vi "ReadExcel.vi"(1 "读出文本":bool, 2 "导出sheet位号":i8=1, 3 "路径":path) -> (0 "EXCEL读取":string[][](array[string]))   [LabVIEW 2011]
panel:
  in  "Excel._Worksheet":refnum<k7>
  in  "Excel._Application":refnum<k7>
  # "将对应路径 Excel 中的表格数据转换为数组数据"
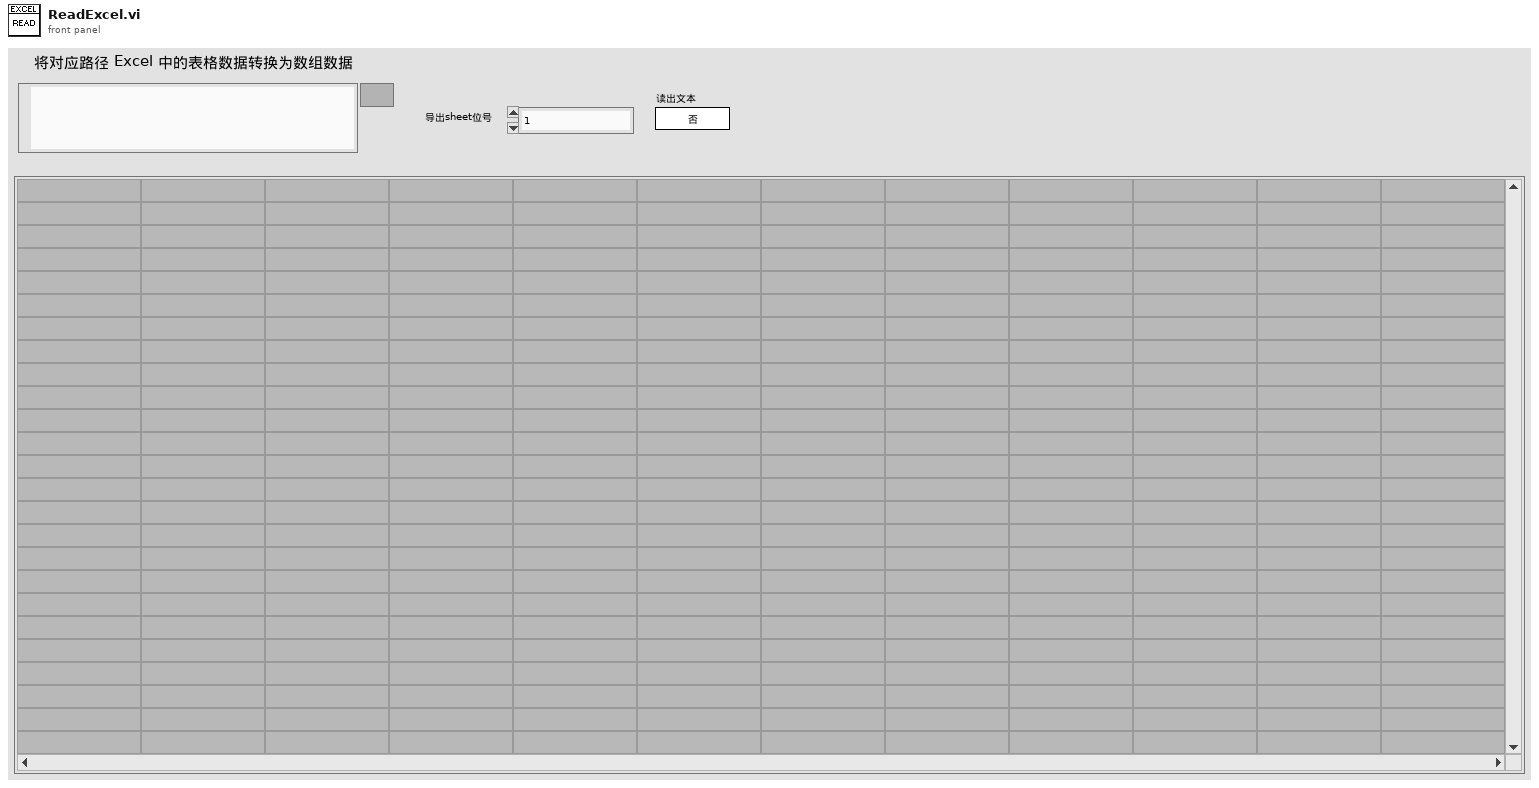
[diagram p1: front panel]
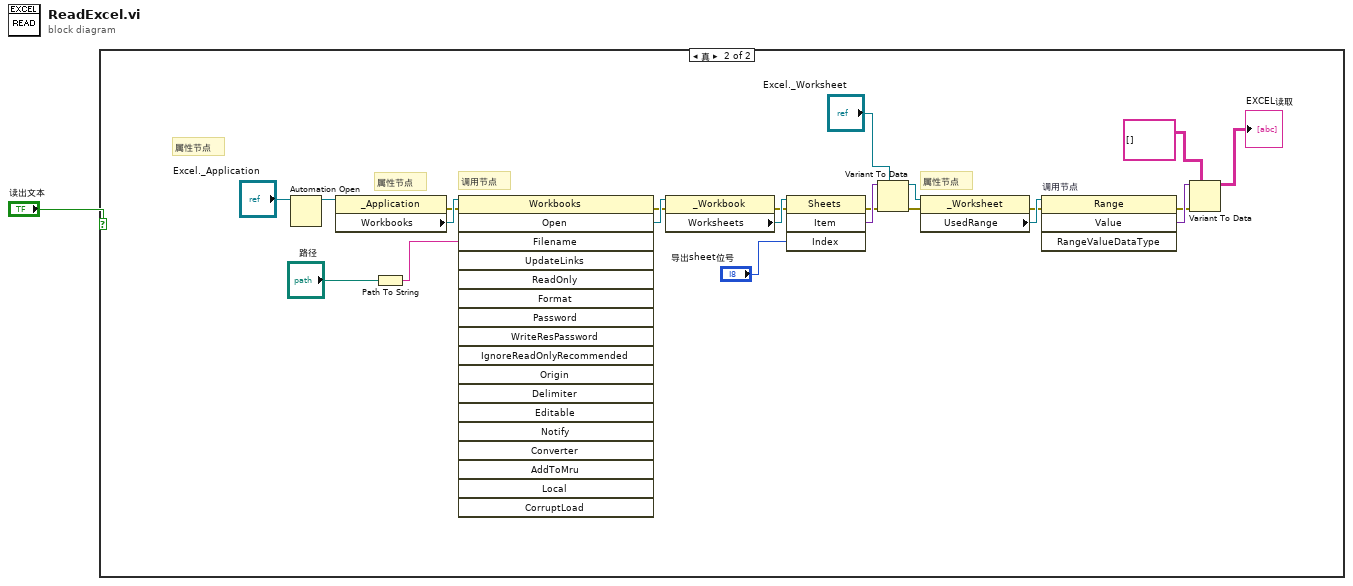
[diagram p0: block diagram]
diagram:
  n1 = case shown="真" "读出文本" {
    frame False {
    }
    frame True {
      # "属性节点"
      # "属性节点"
      # "属性节点"
      # "调用节点"
      n2 = Automation Open(Automation Refnum="Excel._Application") -> (Automation Refnum=w21:refnum<k7>)  [unwired: 3 in, 1 out]
      n3 = property class="_Application"(reference=w21) -> (error out=w19:errorcluster, "Workbooks"=w20:refnum<k7>)  [unwired: 1 in, 1 out]
      n4 = Path To String(path="路径") -> (string=w2:string)
      n5 = invoke class="Workbooks" method="Open"(reference=w20, error in=w19, "Filename"=w2) -> (error out=w17:errorcluster, "Open"=w18:refnum<k7>)  [unwired: 15 in, 16 out]
      n6 = property class="_Workbook"(reference=w18, error in=w17) -> (error out=w14:errorcluster, "Worksheets"=w15:refnum<k7>)  [unwired: 1 out]
      n7 = invoke class="Sheets" method="Item"(reference=w15, error in=w14, "Index"="导出sheet位号") -> (error out=w12:errorcluster, "Item"=w13:variant)  [unwired: 1 in, 2 out]
      n8 = Variant To Data(error in=w12, type="Excel._Worksheet", Variant=w13) -> (data=w10:refnum<k7>, error out=w9:errorcluster)
      n9 = property class="_Worksheet"(reference=w10, error in=w9) -> (error out=w7:errorcluster, "UsedRange"=w8:refnum<k7>)  [unwired: 1 out]
      n10 = invoke on="调用节点" class="Range" method="Value"(reference=w8, error in=w7) -> (error out=w5:errorcluster, "Value"=w6:variant)  [unwired: 2 in, 2 out]
      n11 = Variant To Data(error in=w5, type=string[][] [], Variant=w6) -> (data=→"EXCEL读取":string[][])  [unwired: 1 out]
    }
  }
